vi "TDM Transmit Test.vi"(9 "input valid":bool, 10 "transfer length":u8=32, 11 "sample":u32) -> (1 "ready for input":bool)   [LabVIEW 2013]
uses:
  Source/Controls/i2s signals.ctl
  <vilib>/Platform/TimedLoop/XDataNode/timing_clust.ctl
  <vilib>/Platform/TimedLoop/XDataNode/nitl_modes.ctl
  <vilib>/Platform/TimedLoop/XDataNode/wakeup.ctl
  Source/Controls/tdm configuration.ctl
  <vilib>/rvi/Emulation/niFpgaSctlEmulationGetInTimedLoop.vi
  <vilib>/rvi/Emulation/niFpgaEmulationReportErrorSimple.vi
  <vilib>/rvi/Emulation/niFpgaGetClockAttributes.vi
  <vilib>/rvi/Emulation/niFpgaCriticalErrorInLSC.vi
  <vilib>/Platform/TimedLoop/XDataNode/XDataNode.xnode
  <vilib>/Platform/TimedLoop/XDataNode/XDNodeRunTimeDep.lvlib
  Source/I2S-TDM.lvlib
panel:
  in  "transmit":bool
  out "signals out":T1
  in  "channel count":u8=2
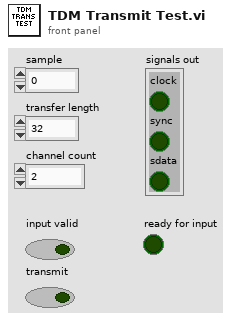
[diagram p1: front panel]
types:
  T1 = typedef "I2S-TDM.lvlib/i2s signals.ctl" = cluster{"clock":bool, "sync":bool, "sdata":bool}
  T2 = typedef "XDNodeRunTimeDep.lvlib/timing_clust.ctl" = cluster{"Expected End [f-1]":u64, "Actual End [f-1]":u64, "Finished Late? [f-1]":bool, "Expected End [i-1]":u64, "Actual End [i-1]":u64, "Finished Late? [i-1]":bool, "Expected Start [i]":u64, "Actual Start [i]":u64, "Expected Start [f]":u64, "Actual Start [f]":u64, "Source Name":string, "Structure Name":string, "Period":i64, "Deadline":i64, "Offset":i64, "Start":i64, "Priority":i32, "Timeout":i32, "Mode":T3, "Wakeup Reason":T4, "Error":errorcluster, "Source Type":string, "Secondary Source Type":string, "Global End Time":u64, "Global Start Time":u64, "Frame Duration":u64, "Iteration Duration":u64, "Assigned CPU":i32, "I/O Scan Engine Mode":u32}
  T3 = typedef "XDNodeRunTimeDep.lvlib/nitl_modes.ctl" = enum32{"No Change", "Process missed periods, maintain original phase", "Discard missed periods, maintain original phase", "Process missed periods, ignore original phase", "Discard missed periods, ignore original phase"}
  T4 = typedef "XDNodeRunTimeDep.lvlib/wakeup.ctl" = enum32{"Normal", "Aborted", "Asynchronous wakeup", "Timing source error", "Timed loop error", "Timeout"}
  T5 = typedef "I2S-TDM.lvlib/tdm configuration.ctl" = cluster{"Number of Channels":u8, "Bits Per Channel":u8, "Bit Set Edge":enum16{"rising", "falling"}, "Invert Frame Sync":bool}
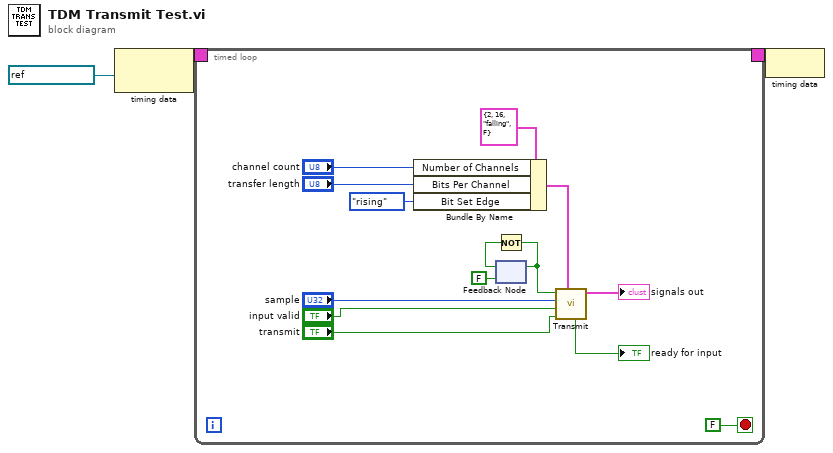
[diagram p0: block diagram]
diagram:
  n1 = node-c288(refnum<k21> "24.576MHz" ("Source Name")) -> (w3:T2)
  n2 = timed-loop {
    timing: w3 -> [_]
    timing-out: [_] -> w2
    stop <- FALSE stop-if-true
    n3 = Bundle By Name(cluster=T5 {"Number of Channels"=2, "Bits Per Channel"=16, "Bit Set Edge"=enum."falling", "Invert Frame Sync"=FALSE} ("Configuration"), "Number of Channels"="channel count", "Bits Per Channel"="transfer length", "Bit Set Edge"=enum16{"rising", "falling"}."rising") -> (w9:T5)
    n4 = feedback #1(FALSE) -> (w16:bool)
    n5 = Not(x=w16) -> (.not. x?=w15:bool)
    n6 = feedback-in #1(w15) -> ()
    n7 = call "Transmit.vi"("configuration"=w9, "transmit"="transmit", "input valid"="input valid", "sample"="sample", "clock in"=w15) -> ("signals out"=→"signals out":T1, "ready for input"=→"ready for input":bool)  [unwired: 5 in]
  }
  n8 = node-c288(w2) -> ()
